vi "Measurement Type.vi"(8 "error in (no error)":errorcluster, 10 "Settings":T1, 11 "UI":refnum<queue>) -> (0 "error out":errorcluster)   [LabVIEW 2014, in "AvaSpec.lvlib" / "AvaSpec Acquisition.lvlib"]
uses:
  AvaSpec Acquisition.lvlib
  Settings/Settings.ctl
  Hardware Configuration.ctl
  Libraries/AS-5216-DLL/AVS settings.ctl
  Sphere Indicator.ctl
  Settings/Measurement Type.ctl
  Logging/Logging Configuration.ctl
  support/Message Queue/Message Cluster.ctl
  support/Message Queue/Enqueue Message (Single).vi
  support/Message Queue/AvaSpec Message Queue.lvlib
  Dark/Dark.lvlib
  AvaSpec.lvlib
  Logging/AvaSpec Logging.lvlib
  Settings/AvaSpec Settings.lvlib
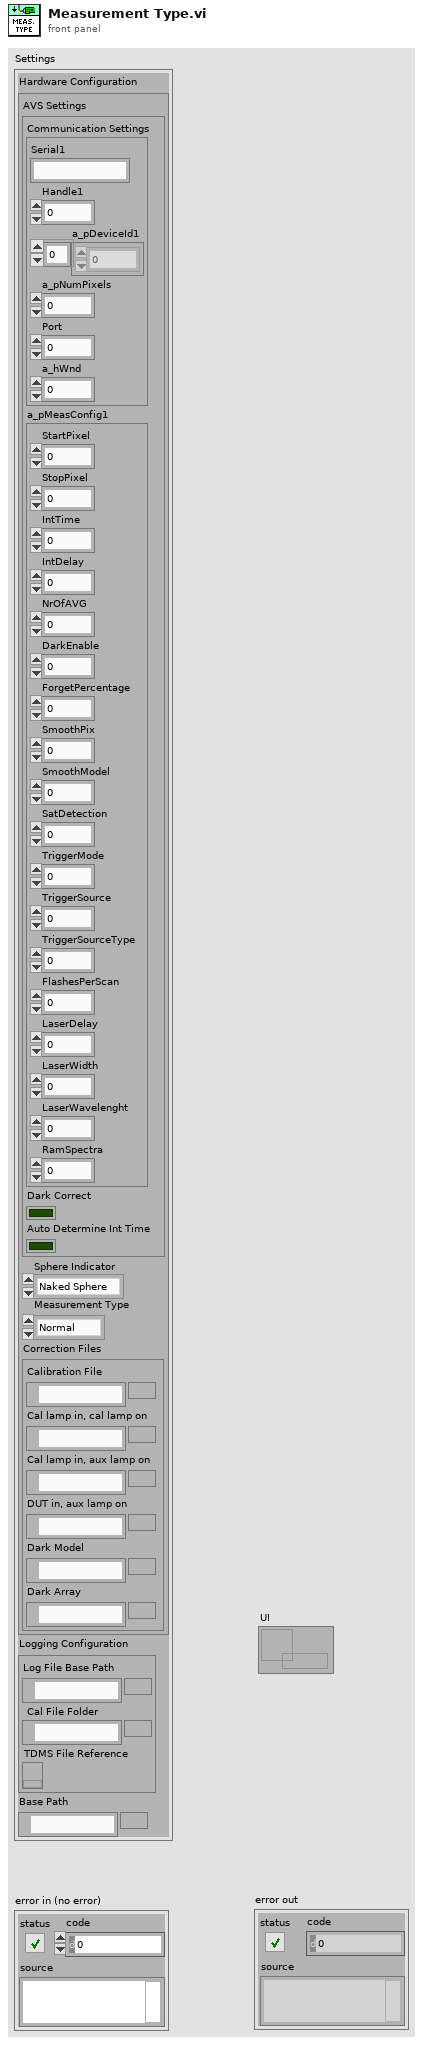
[diagram p1: front panel]
types:
  T1 = typedef "AvaSpec.lvlib/AvaSpec Settings.lvlib/Settings.ctl" = cluster{"Hardware Configuration":T2, "Logging Configuration":T6, "Base Path":path}
  T2 = typedef "AvaSpec.lvlib/AvaSpec Acquisition.lvlib/Hardware Configuration.ctl" = cluster{"AVS Settings":T3, "Sphere Indicator":T4, "Measurement Type":T5, "Correction Files":cluster{"Calibration File":path, "Cal lamp in, cal lamp on":path, "Cal lamp in, aux lamp on":path, "DUT in, aux lamp on":path, "Dark Model":path, "Dark Array":path}}
  T3 = typedef "AvaSpec.lvlib/AVS settings.ctl" = cluster{"Communication Settings":cluster{"Serial1":string, "Handle1":i32, "a_pDeviceId1":u8[], "a_pNumPixels":u16, "Port":i32, "a_hWnd":i32}, "a_pMeasConfig1":cluster{"StartPixel":u16, "StopPixel":u16, "IntTime":sgl, "IntDelay":u32, "NrOfAVG":u32, "DarkEnable":u8, "ForgetPercentage":u8, "SmoothPix":u16, "SmoothModel":u8, "SatDetection":u8, "TriggerMode":u8, "TriggerSource":u8, "TriggerSourceType":u8, "FlashesPerScan":u16, "LaserDelay":u32, "LaserWidth":u32, "LaserWavelenght":sgl, "RamSpectra":u16}, "Dark Correct":bool, "Auto Determine Int Time":bool}
  T4 = typedef "AvaSpec.lvlib/Sphere Indicator.ctl" = enum16{"Naked Sphere", "Insulated Sphere"}
  T5 = typedef "AvaSpec.lvlib/AvaSpec Acquisition.lvlib/Measurement Type.ctl" = enum16{"Normal", "Calibration", "Dark"}
  T6 = typedef "AvaSpec.lvlib/AvaSpec Logging.lvlib/Logging Configuration.ctl" = cluster{"Log File Base Path":path, "Cal File Folder":path, "TDMS File Reference":refnum<k34>}
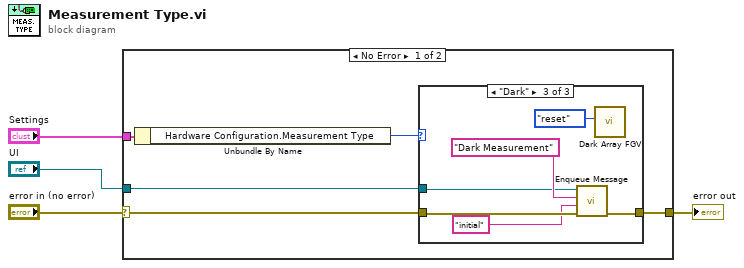
[diagram p0: block diagram]
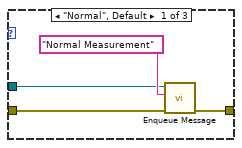
[diagram p2: hidden frame]
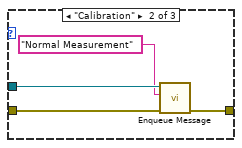
[diagram p3: hidden frame]
diagram:
  n1 = case shown="No Error" "error in (no error)" {
    selector: "error in (no error)" -> [w6 w24]
    tunnel: "Settings" -> [w9 _]
    tunnel: [w5 w24] -> w2
    tunnel: "UI" -> [w7 _]
    frame No Error {
      n2 = Unbundle By Name(w9) -> ("Hardware Configuration.Measurement Type"=w8:T5)
      n3 = case shown="\"Dark\"" w8 {
        tunnel: w7 -> [w12 w17 w22]
        tunnel: w6 -> [w11 w15 w21]
        tunnel: [w10 w14 w20] -> w5
        frame "Normal", Default {
          n4 = call-poly "Enqueue Message.vi"("error in (no error)"=w11, "Message"="Normal Measurement", "Message Queue"=w12) -> ("error out"=w10:errorcluster)  [unwired: 7 in, 1 out]
        }
        frame "Calibration" {
          n5 = call-poly "Enqueue Message.vi"("error in (no error)"=w15, "Message"="Normal Measurement", "Message Queue"=w17) -> ("error out"=w14:errorcluster)  [unwired: 7 in, 1 out]
        }
        frame "Dark" {
          n6 = call-poly "Enqueue Message.vi"("error in (no error)"=w21, "Message Data"="initial" ("Message"), "Message"="Dark Measurement", "Message Queue"=w22) -> ("error out"=w20:errorcluster)  [unwired: 6 in, 1 out]
          n7 = call "Dark Array FGV.vi"("Control"=enum16{"get", "add", "reset"}."reset") -> ()  [unwired: 10 in, 1 out]
        }
      }
    }
    frame Error {
    }
  }
  "error out" <- w2
